vi "BRig_Host__Loop_Consumer_RunState__getType.vi"(11 "input_strCmd":string) -> (2 "output_RunState_type":u8)   [LabVIEW 2014]
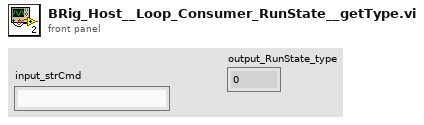
[diagram p1: front panel]
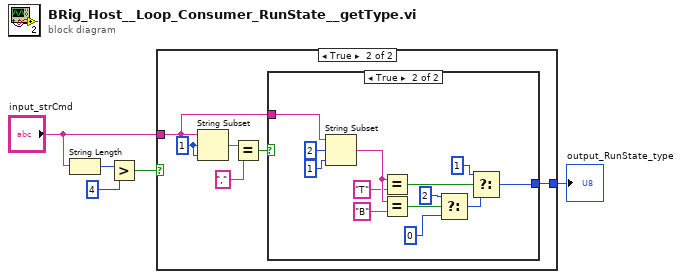
[diagram p0: block diagram]
diagram:
  n1 = String Length(string="input_strCmd") -> (length=w5:i32)
  n2 = Greater?(x=w5, y=4) -> (0:w3:bool)
  n3 = case shown="True" w3 {
    tunnel: "input_strCmd" -> [_ w7]
    tunnel: [_ w6] -> w1
    frame False {
    }
    frame True {
      w11 = 1 ("offset (0)")
      n4 = String Subset(string=w7, offset (0)=w11, length (rest)=w11) -> (substring=w9:string)
      n5 = Equal?(x=w9, y=",") -> (x = y?=w8:bool)
      n6 = case shown="True" w8 {
        tunnel: w7 -> [_ w23]
        tunnel: [_ w12] -> w6
        frame False {
        }
        frame True {
          n7 = String Subset(string=w23, offset (0)=2, length (rest)=1 ("offset (0)")) -> (substring=w21:string)
          n8 = Equal?(x=w21, y="T") -> (x = y?=w14:bool)
          n9 = Equal?(x=w21, y="B") -> (x = y?=w18:bool)
          n10 = Select(t=u8 2, s=w18, f=u8 0 ("offset (0)")) -> (s? t:f=w13:u8)
          n11 = Select(t=u8 1, s=w14, f=w13) -> (s? t:f=w12:u8)
        }
      }
    }
  }
  "output_RunState_type" <- w1
